vi "Set Delay After Transaction.vi"(8 "error in (no error)":errorcluster, 10 "delay, ms":u32, 11 "MODBUS in":refnum<class "Modbus.lvclass">) -> (0 "error out":errorcluster, 3 "MODBUS Out":refnum<class "Modbus.lvclass">)   [LabVIEW 2020, in "Library Instrument & Equipement.lvlib" / "Library Relay_Board.lvlib" / "Modbus.lvclass"]
doc: "Sets delay after transaction. This can be useful when RS-485 device is slow to release the interface."
uses:
  Modbus.lvclass
  Modbus.lvclass/Modbus.ctl
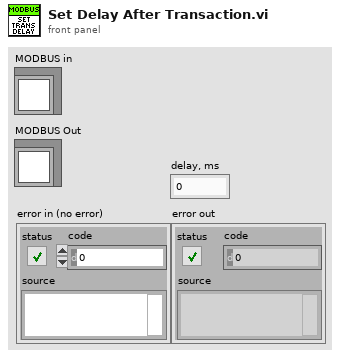
[diagram p1: front panel]
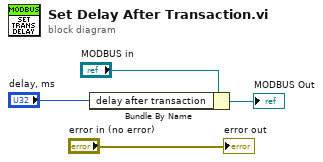
[diagram p0: block diagram]
diagram:
  n1 = Bundle By Name(cluster="MODBUS in", "delay after transaction"="delay, ms") -> (→"MODBUS Out":refnum<class "Modbus.lvclass">)
  "error out" <- "error in (no error)"
